vi "String to Hex.vi"(11 "body":string) -> (3 "hex string":string)   [LabVIEW 2015]
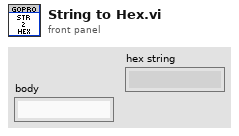
[diagram p1: front panel]
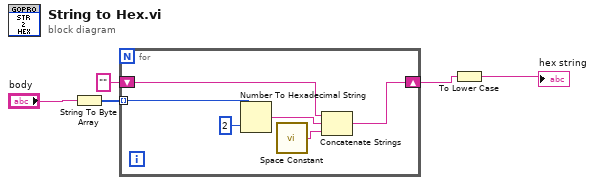
[diagram p0: block diagram]
diagram:
  n1 = String To Byte Array(string="body") -> (unsigned byte array=w5:u8[])
  n2 = for {
    tunnel: w5 -> [w11] mode=indexing
    shift-right: [w8] -> w2
    shift-left: "" -> [w7]
    n3 = Number To Hexadecimal String(1:i16 2 ("width (-)"), 2:w11) -> (0:w10:string)
    n4 = call <vilib>:"Space Constant.vi"() -> ("String"=w9:string)
    n5 = Concatenate Strings(w7, w10, w9) -> (w8:string)
  }
  n6 = To Lower Case(string=w2) -> (all lower case string=→"hex string":string)
